vi "Reset Gyro.vi"(11 "Gyro ID (1 or 2)":i32) -> ()   [LabVIEW 2013]
uses:
  Gyro Global.vi
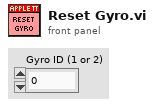
[diagram p1: front panel]
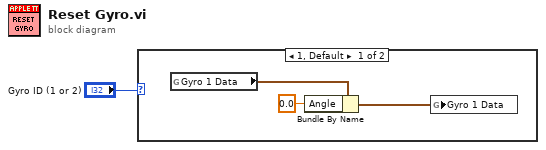
[diagram p0: block diagram]
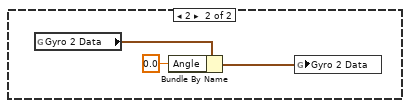
[diagram p2: hidden frame]
diagram:
  n1 = case shown="1, Default" "Gyro ID (1 or 2)" {
    frame 1, Default {
      n2 = global read "Gyro Global.vi" "Gyro 1 Data"() -> (w3:cluster{"Rate":dbl, "Angle":dbl, "Gain":dbl})
      n3 = Bundle By Name(cluster=w3, "Angle"=0.0) -> (w2:cluster{"Rate":dbl, "Angle":dbl, "Gain":dbl})
      n4 = global write "Gyro Global.vi" "Gyro 1 Data"(w2) -> ()
    }
    frame 2 {
      n5 = global read "Gyro Global.vi" "Gyro 2 Data"() -> (w6:cluster{"Rate":dbl, "Angle":dbl, "Gain":dbl})
      n6 = Bundle By Name(cluster=w6, "Angle"=0.0) -> (w5:cluster{"Rate":dbl, "Angle":dbl, "Gain":dbl})
      n7 = global write "Gyro Global.vi" "Gyro 2 Data"(w5) -> ()
    }
  }
